vi "Write Format String.vi"(5 "Format String":string, 9 "NumericText in":refnum<class "Digital.lvclass">) -> (3 "NumericText out":refnum<class "Digital.lvclass">)   [LabVIEW 2014, in "Digital.lvclass"]
uses:
  Digital.lvclass
  Digital.lvclass/Digital.ctl
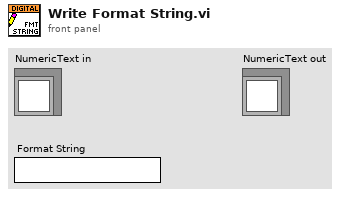
[diagram p1: front panel]
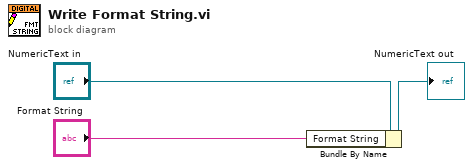
[diagram p0: block diagram]
diagram:
  n1 = Bundle By Name(cluster="NumericText in", "Format String"="Format String") -> (→"NumericText out":refnum<class "Digital.lvclass">)
